vi "Create_Object.vi"(8 "error in (no error)":errorcluster, 9 "Terminal Map in":map{string, T1}(c390), 10 "vi refnum in":refnum<vi>, 11 "Numeric Constant in":refnum<class "Numeric Constant.lvclass">) -> (0 "error out":errorcluster, 1 "Terminal Map Out":map{string, T1}(c390), 3 "Numeric Constant out":refnum<class "Numeric Constant.lvclass">)   [LabVIEW 2025, in "Numeric Constant.lvclass"]
uses:
  Numeric Constant.lvclass
  home/jake/Documents/github/LVGPT/LabVIEW/VIs/Classes/Node/Node.lvclass
  Terminal.ctl
  <vilib>/numeric/LVNumericRepresentation.ctl
  Node.lvclass/Node.ctl
  Constant.lvclass
  Node.lvclass
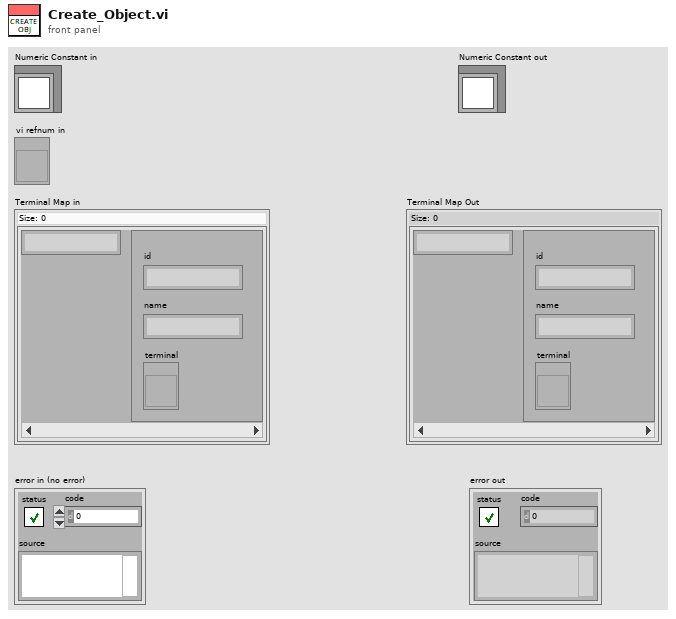
[diagram p1: front panel]
types:
  T1 = typedef "Terminal.ctl" = cluster{"id":string, "name":string, "terminal":refnum<vi>}
  T2 = typedef "LVNumericRepresentation.ctl" = enum32{"Extended Precision", "Double Precision", "Single Precision", "Long", "Word", "Byte", "Unsigned Long", "Unsigned Word", "Unsigned Byte", "Complex Extended", "Complex Double", "Complex Single", "Quad", "Unsigned Quad", "Fixed-Point"}
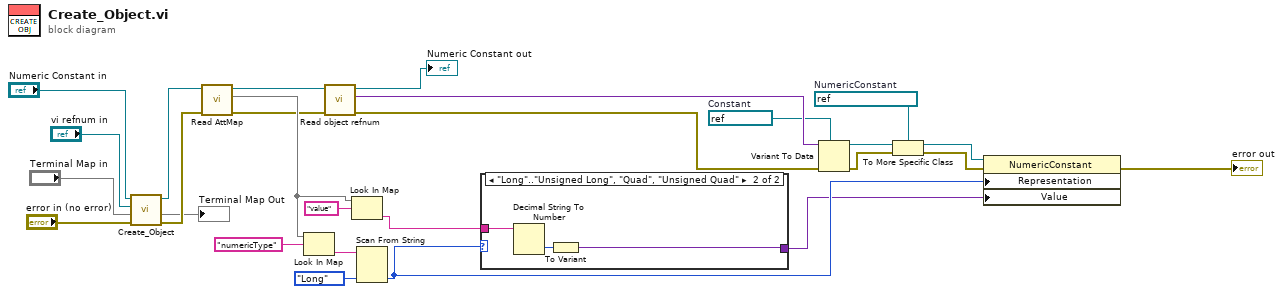
[diagram p0: block diagram]
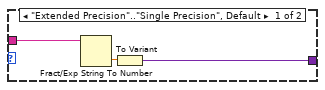
[diagram p2: hidden frame]
diagram:
  w5 = refnum<vi> refnum  # NumericConstant
  w11 = refnum<vi> refnum  # Constant
  n1 = call-parent "Create_Object.vi"("error in (no error)"="error in (no error)", "Terminal Map in"="Terminal Map in", "vi refnum in"="vi refnum in", "Constant in"="Numeric Constant in") -> ("error out"=w15:errorcluster, "Terminal Map Out"=→"Terminal Map Out":map{string, T1}, "Constant out"=w20:refnum<class "Numeric Constant.lvclass">)  [unwired: 5 in]
  n2 = call "Read AttMap.vi"("error in (no error)"=w15, "Node in"=w20) -> ("error out"=w13:errorcluster, "AttMap"=w18:map{string, string}, "Node out"=w16:refnum<class "Numeric Constant.lvclass">)  [unwired: 7 in]
  n3 = Look In Map(map=w18, key="numericType") -> (value=w21:string)  [unwired: 1 in, 1 out]
  n4 = call-dynamic "Read object refnum.vi"("error in (no error)"=w13, "Node in"=w16) -> ("error out"=w9:errorcluster, "object refnum"=w12:variant, "Node out"=→"Numeric Constant out":refnum<class "Numeric Constant.lvclass">)  [unwired: 7 in]
  n5 = Look In Map(map=w18, key="value") -> (value=w17:string)  [unwired: 1 in, 1 out]
  n6 = Scan From String(input string=w21, default 1=LVNumericRepresentation."Long" ("Representation")) -> (output 1=w2:T2)  [unwired: 3 in, 3 out]
  n7 = case shown="\"Long\"..\"Unsigned Long\", \"Quad\", \"Unsigned Quad\"" w2 {
    tunnel: w17 -> [w30 w33]
    tunnel: [w28 w31] -> w1
    frame "Extended Precision".."Single Precision", Default {
      n8 = Fract/Exp String To Number(string=w30) -> (number=w29:dbl)  [unwired: 3 in, 1 out]
      n9 = To Variant(anything=w29) -> (Variant=w28:variant)
    }
    frame "Long".."Unsigned Long", "Quad", "Unsigned Quad" {
      n10 = Decimal String To Number(string=w33) -> (number=w32:i32)  [unwired: 2 in, 1 out]
      n11 = To Variant(anything=w32) -> (Variant=w31:variant)
    }
  }
  n12 = Variant To Data(error in=w9, type=w11, Variant=w12) -> (data=w10:refnum<vi>, error out=w4:errorcluster)
  n13 = To More Specific Class(target class=w5, reference=w10, error in=w4) -> (specific class reference=w6:refnum<vi>, error out=w3:errorcluster)
  n14 = property class="NumericConstant"(reference=w6, error in=w3, "Representation"=w2, "Value"=w1) -> (error out=→"error out":errorcluster)  [unwired: 1 out]
